vi "formal.vi"() -> ()   [LabVIEW 2011]
uses:
  <vilib>/Platform/storage/lvStorage.llb/_openFunction.ctl
  <vilib>/DAQmx/read.llb/DAQmx Read (Analog 1D Wfm NChan NSamp).vi
  <vilib>/Utility/file.llb/Write To Spreadsheet File (string).vi
  <vilib>/DAQmx/configure/timing.llb/DAQmx Timing (Sample Clock).vi
  <vilib>/Waveform/WDTOps.llb/WDT Index Channel DBL.vi
  <vilib>/Platform/storage/lvStorage.llb/_openStorageWithRootAutoDetect.vi
  <vilib>/Platform/storage/lvStorage.llb/xStorage/xStorageSupp/ErrorOut.vi
  <vilib>/Platform/storage/lvStorage.llb/_queryPropDateTime.vi
  <vilib>/Platform/storage/lvStorage.llb/_queryGenericObjects.vi
  <vilib>/Platform/storage/lvStorage.llb/_loadAllWaveform.vi
  <vilib>/Platform/storage/Storage.llb/Get Object Info.vi
  <vilib>/Platform/storage/Storage.llb/__closeStorageFromObject.vi
  <vilib>/DAQmx/calibration/calibrationInfo.llb/DAQmx Perform Shunt Calibration (Strain).vi
  <vilib>/DAQmx/miscellaneous.llb/DAQmx Fill In Error Info.vi
  <vilib>/Utility/file.llb/Write To Spreadsheet File (DBL).vi
  <vilib>/Platform/storage/lvStorage.llb/xStorage/Open Data Storage/Open Data Storage.xnode
  <vilib>/Platform/storage/lvStorage.llb/xStorage/Read Data/Read Data.xnode
  <vilib>/Platform/storage/lvStorage.llb/xStorage/Close Data Storage/Close Data Storage.xnode
  C:/Program Files (x86)/National Instruments/LabVIEW 2011/resource/objmgr/daqmx.rc
  <vilib>/Analysis/NI_AALBase.lvlib
panel:
  out "Working Folder":string="M:\\github\\DAQP"
  out "concatenated string":string="M:\\github\\DAQP\\_SP11_file_0.tdms"
  in  "stop":bool
  in  "voltage excitation source 2":i32(ring)=10200 items=["Internal"=10200, "External"=10167, "None"=10230]
  in  "voltage excitation source":i32(ring)=10200 items=["Internal"=10200, "External"=10167, "None"=10230]
  out "Config Flat Array":T1(array[cluster])=[{["234", "VoltageInputIntExc", "SC1mod1/ai0", "LVDT_5", "in."], "Voltage_cluster"={10.0, -10.0, 22.4, 0.0, TRUE, 60.0, 10.0}, "Strain_cluster"={0.0, 0.0, 0.0, 0.0, TRUE, 0.0, 0.0, 0.0, 0.0, ""}}, {["234424", "VoltageInputExtExc", "SC1mod1/ai1", "MTS_DISP_0_10_in", "in."], "Voltage_cluster"={10.0, -10.0, 22.4, 0.0, TRUE, 60.0, 0.4}, "Strain_cluster"={0.0, 0.0, 0.0, 0.0, TRUE, 0.0, 0.0, 0.0, 0.0, ""}}, {["1234", "StrainInput", "SC1mod1/ai2", "STRAIN_350_half", "microstrain"], "Voltage_cluster"={0.0, 0.0, 0.0, 0.0, TRUE, 0.0, 0.0}, "Strain_cluster"={0.01, -0.01, 1.0, 0.0, TRUE, 60.0, 3.125, 350.0, 2.0, "Half Bridge I"}}]
  out "Channel Indicator":i32[](array[numeric])=[2, 1, 0]
  out "Config Array":T1(array[cluster])=[{["234", "VoltageInputIntExc", "SC1mod1/ai0", "LVDT_5", "in."], "Voltage_cluster"={10.0, -10.0, 22.4, 0.0, TRUE, 60.0, 10.0}, "Strain_cluster"={0.0, 0.0, 0.0, 0.0, TRUE, 0.0, 0.0, 0.0, 0.0, ""}}, {["234424", "VoltageInputExtExc", "SC1mod1/ai1", "MTS_DISP_0_10_in", "in."], "Voltage_cluster"={10.0, -10.0, 22.4, 0.0, TRUE, 60.0, 0.4}, "Strain_cluster"={0.0, 0.0, 0.0, 0.0, TRUE, 0.0, 0.0, 0.0, 0.0, ""}}, {["1234", "StrainInput", "SC1mod1/ai2", "STRAIN_350_half", "microstrain"], "Voltage_cluster"={0.0, 0.0, 0.0, 0.0, TRUE, 0.0, 0.0}, "Strain_cluster"={0.01, -0.01, 1.0, 0.0, TRUE, 60.0, 3.125, 350.0, 2.0, "Half Bridge I"}}, {[], "Voltage_cluster"={0.0, 0.0, 0.0, 0.0, TRUE, 0.0, 0.0}, "Strain_cluster"={0.0, 0.0, 0.0, 0.0, TRUE, 0.0, 0.0, 0.0, 0.0, ""}}, {[], "Voltage_cluster"={0.0, 0.0, 0.0, 0.0, TRUE, 0.0, 0.0}, "Strain_cluster"={0.0, 0.0, 0.0, 0.0, TRUE, 0.0, 0.0, 0.0, 0.0, ""}}, {[], "Voltage_cluster"={0.0, 0.0, 0.0, 0.0, TRUE, 0.0, 0.0}, "Strain_cluster"={0.0, 0.0, 0.0, 0.0, TRUE, 0.0, 0.0, 0.0, 0.0, ""}}, {[], "Voltage_cluster"={0.0, 0.0, 0.0, 0.0, TRUE, 0.0, 0.0}, "Strain_cluster"={0.0, 0.0, 0.0, 0.0, TRUE, 0.0, 0.0, 0.0, 0.0, ""}}, {[], "Voltage_cluster"={0.0, 0.0, 0.0, 0.0, TRUE, 0.0, 0.0}, "Strain_cluster"={0.0, 0.0, 0.0, 0.0, TRUE, 0.0, 0.0, 0.0, 0.0, ""}}, {[], "Voltage_cluster"={0.0, 0.0, 0.0, 0.0, TRUE, 0.0, 0.0}, "Strain_cluster"={0.0, 0.0, 0.0, 0.0, TRUE, 0.0, 0.0, 0.0, 0.0, ""}}, {[], "Voltage_cluster"={0.0, 0.0, 0.0, 0.0, TRUE, 0.0, 0.0}, "Strain_cluster"={0.0, 0.0, 0.0, 0.0, TRUE, 0.0, 0.0, 0.0, 0.0, ""}}, {[], "Voltage_cluster"={0.0, 0.0, 0.0, 0.0, TRUE, 0.0, 0.0}, "Strain_cluster"={0.0, 0.0, 0.0, 0.0, TRUE, 0.0, 0.0, 0.0, 0.0, ""}}, {[], "Voltage_cluster"={0.0, 0.0, 0.0, 0.0, TRUE, 0.0, 0.0}, "Strain_cluster"={0.0, 0.0, 0.0, 0.0, TRUE, 0.0, 0.0, 0.0, 0.0, ""}}, {[], "Voltage_cluster"={0.0, 0.0, 0.0, 0.0, TRUE, 0.0, 0.0}, "Strain_cluster"={0.0, 0.0, 0.0, 0.0, TRUE, 0.0, 0.0, 0.0, 0.0, ""}}, {[], "Voltage_cluster"={0.0, 0.0, 0.0, 0.0, TRUE, 0.0, 0.0}, "Strain_cluster"={0.0, 0.0, 0.0, 0.0, TRUE, 0.0, 0.0, 0.0, 0.0, ""}}, {[], "Voltage_cluster"={0.0, 0.0, 0.0, 0.0, TRUE, 0.0, 0.0}, "Strain_cluster"={0.0, 0.0, 0.0, 0.0, TRUE, 0.0, 0.0, 0.0, 0.0, ""}}, {[], "Voltage_cluster"={0.0, 0.0, 0.0, 0.0, TRUE, 0.0, 0.0}, "Strain_cluster"={0.0, 0.0, 0.0, 0.0, TRUE, 0.0, 0.0, 0.0, 0.0, ""}}, {[], "Voltage_cluster"={0.0, 0.0, 0.0, 0.0, TRUE, 0.0, 0.0}, "Strain_cluster"={0.0, 0.0, 0.0, 0.0, TRUE, 0.0, 0.0, 0.0, 0.0, ""}}, {[], "Voltage_cluster"={0.0, 0.0, 0.0, 0.0, TRUE, 0.0, 0.0}, "Strain_cluster"={0.0, 0.0, 0.0, 0.0, TRUE, 0.0, 0.0, 0.0, 0.0, ""}}, {[], "Voltage_cluster"={0.0, 0.0, 0.0, 0.0, TRUE, 0.0, 0.0}, "Strain_cluster"={0.0, 0.0, 0.0, 0.0, TRUE, 0.0, 0.0, 0.0, 0.0, ""}}, {[], "Voltage_cluster"={0.0, 0.0, 0.0, 0.0, TRUE, 0.0, 0.0}, "Strain_cluster"={0.0, 0.0, 0.0, 0.0, TRUE, 0.0, 0.0, 0.0, 0.0, ""}}, {[], "Voltage_cluster"={0.0, 0.0, 0.0, 0.0, TRUE, 0.0, 0.0}, "Strain_cluster"={0.0, 0.0, 0.0, 0.0, TRUE, 0.0, 0.0, 0.0, 0.0, ""}}, {[], "Voltage_cluster"={0.0, 0.0, 0.0, 0.0, TRUE, 0.0, 0.0}, "Strain_cluster"={0.0, 0.0, 0.0, 0.0, TRUE, 0.0, 0.0, 0.0, 0.0, ""}}, {[], "Voltage_cluster"={0.0, 0.0, 0.0, 0.0, TRUE, 0.0, 0.0}, "Strain_cluster"={0.0, 0.0, 0.0, 0.0, TRUE, 0.0, 0.0, 0.0, 0.0, ""}}, {[], "Voltage_cluster"={0.0, 0.0, 0.0, 0.0, TRUE, 0.0, 0.0}, "Strain_cluster"={0.0, 0.0, 0.0, 0.0, TRUE, 0.0, 0.0, 0.0, 0.0, ""}}, {[], "Voltage_cluster"={0.0, 0.0, 0.0, 0.0, TRUE, 0.0, 0.0}, "Strain_cluster"={0.0, 0.0, 0.0, 0.0, TRUE, 0.0, 0.0, 0.0, 0.0, ""}}, {[], "Voltage_cluster"={0.0, 0.0, 0.0, 0.0, TRUE, 0.0, 0.0}, "Strain_cluster"={0.0, 0.0, 0.0, 0.0, TRUE, 0.0, 0.0, 0.0, 0.0, ""}}, {[], "Voltage_cluster"={0.0, 0.0, 0.0, 0.0, TRUE, 0.0, 0.0}, "Strain_cluster"={0.0, 0.0, 0.0, 0.0, TRUE, 0.0, 0.0, 0.0, 0.0, ""}}, {[], "Voltage_cluster"={0.0, 0.0, 0.0, 0.0, TRUE, 0.0, 0.0}, "Strain_cluster"={0.0, 0.0, 0.0, 0.0, TRUE, 0.0, 0.0, 0.0, 0.0, ""}}, {[], "Voltage_cluster"={0.0, 0.0, 0.0, 0.0, TRUE, 0.0, 0.0}, "Strain_cluster"={0.0, 0.0, 0.0, 0.0, TRUE, 0.0, 0.0, 0.0, 0.0, ""}}, {[], "Voltage_cluster"={0.0, 0.0, 0.0, 0.0, TRUE, 0.0, 0.0}, "Strain_cluster"={0.0, 0.0, 0.0, 0.0, TRUE, 0.0, 0.0, 0.0, 0.0, ""}}, {[], "Voltage_cluster"={0.0, 0.0, 0.0, 0.0, TRUE, 0.0, 0.0}, "Strain_cluster"={0.0, 0.0, 0.0, 0.0, TRUE, 0.0, 0.0, 0.0, 0.0, ""}}, {[], "Voltage_cluster"={0.0, 0.0, 0.0, 0.0, TRUE, 0.0, 0.0}, "Strain_cluster"={0.0, 0.0, 0.0, 0.0, TRUE, 0.0, 0.0, 0.0, 0.0, ""}}]
  in  "Tab Control":T2(tab)=enum."check Fatigue tdms file"
  in  "SXCI Chassis Name":string="/SC1"
  in  "Config File Path":path=path "M:/github/DAQP/xml_temp.xml"
  in  "Task Name":refnum<k21>="new Task"
  in  "custom scale name":tag="linear1"
  in  "error in":errorcluster
  out "Total Number of Channel in Use":i32=3
  in  "Go Button":bool
  out "Utility Usage Array":cluster{bool, string}[][](array[cluster])=[[{TRUE, "234"}, {FALSE, ""}, {FALSE, ""}, {FALSE, ""}], [{TRUE, "234424"}, {FALSE, ""}, {FALSE, ""}, {FALSE, ""}], [{TRUE, "1234"}, {FALSE, ""}, {FALSE, ""}, {FALSE, ""}], [{FALSE, ""}, {FALSE, ""}, {FALSE, ""}, {FALSE, ""}], [{FALSE, ""}, {FALSE, ""}, {FALSE, ""}, {FALSE, ""}], [{FALSE, ""}, {FALSE, ""}, {FALSE, ""}, {FALSE, ""}], [{FALSE, ""}, {FALSE, ""}, {FALSE, ""}, {FALSE, ""}], [{FALSE, ""}, {FALSE, ""}, {FALSE, ""}, {FALSE, ""}]]
  in  "Measure actual excitation?":bool
  in  "Shunt Resistance":dbl=100000.0 format="%0.2f"
  in  "Shunt Location":enum32{"R1", "R2", "R3", "R4"}(ring)=enum."R3"
  in  "error out":errorcluster
  in  "sample rate":dbl=1000.0
  in  "number of samples per channel (buffer size)":i32=10000000
  in  "number of samples per channel":i32=200
  in  "Offset Nulling":bool
  in  "Display Channel":u16(ring)=1 items=["234", "234424", "1234"]
  out "Display Channel results":dbl[](graph)=[22.61393258426966] caption="Real Time Data Acquision Chart"
  out "Result Array":dbl[](array[numeric])=[3.695945285784074, 22.61393258426966, -0.0019209204014080854]
  out "Strain Channel Name":string[](array[string])=["1234"]
  out "Channel Physical Name":string[](array[string])=["SC1mod1/ai0", "SC1mod1/ai1", "SC1mod1/ai2"]
  out "Channel Name Array":string[](array[string])=["234", "234424", "1234"]
  out "Channel Unit Array":string[](array[string])=["in.", "in.", "microstrain"]
  out "Factor A":dbl[](array[numeric])=[22.4, 22.4, 1.0]
  out "Factor B":dbl[](array[numeric])
  out "Factor N":dbl[](array[numeric])
  in  "Start DAQ":bool=TRUE
  in  "shunt":bool
  out "LVM result file path":path=path "M:/github/DAQP/trial_newnew.lvm"
  out "AvailSampPerChan":u32=9
  in  "Start Recording":bool
  out "Csv Result File":path=path "M:/github/DAQP/trial_newnew.txt"
  in  "Record File Path":string="trial_newnew"
  in  "Start Fatigue Module":bool=TRUE
  in  "Recording cycles (M)":i32=5
  in  "Recording interval (N)":i32=10
  out "Cycle count measuring":string="234"
  in  "Name of specimen":string="_SP11"
  in  "Lowerbound":dbl=-4.6
  in  "Upbond":dbl=4.6
  in  "Channel to count cycle":i32
  out "Fatigue data recording in progress":bool=TRUE
  out "Valley":bool
  out "Peak":bool=TRUE
  out "Current cycle numbers":dbl
  in  "Start Cycle":i32
  in  "file path":path=path "C:/Documents and Settings/ju112496/Desktop/seminar/seminar1_SP11_file_30.tdms"
  out "Total Channel numbers":i32=3
  in  "Display channel":i32
  out "Display Channel name":string="potential meter"
  in  "Load file":bool
  out "Waveform Graph":waveform(dbl)(graph)={"t0"=timestamp(3600 s since 1904-01-01), "dt"=1.0, "Y"=[4.96518220736595, 4.9879295957189544, 4.987880843319572, 4.9878564031395225, 4.98785639543025, 4.98785639543025, 4.987880804692245, 4.9878563940215805, 4.9878960256751075, 4.987890269213241, 4.987881073821511, 4.987880252277753, 4.987929618872902, 4.987856395547572, 4.98788080318033, 4.987856395533495, 4.987880803283583, 4.987906295992125, 4.98787971833429, 4.9878586312981446, 4.987878567509733, 4.987856395430245, 4.98785639543025, 4.98785639543025, 4.98785639543025, 4.987883590063237, 4.987878016503915, 4.98788151128357, 4.987855687430249, 4.98785639543025, 4.987929617963517, 4.9878563964569524, 4.987880803283373, 4.987856395430452, 4.98785639543025, 4.98785639543025, 4.98788084098527, 4.987880765581879, 4.987931213533417, 4.987879208800789, 4.987930169857925, 4.987855844502128, 4.987874416787948, 4.987880803283574, 4.987935976028989, 4.9879052089034515, 4.987954058719019, 4.9847496503819215, 2.892462538878111, -2.2229287425946533, -4.973634617887958, -5.002277969332104, -5.0022779693255774, -5.0022779693255774, -5.001646607827787, -0.31893796746551445, 4.632149520376136, 4.98790575411758, 4.98792911085913, 4.9878808211186305, 4.98788080338445, 4.987929900245035, 4.987904929884249, 4.698784785906143, 0.9667412484497627, -3.879258099878396, -5.002259664842451, -5.00227796932558, -5.0022779693255774, -5.0022779693255774, -5.0022779693255774, -1.4532621065694493, 4.4686316784738045, 4.987856401837168, 4.987905209618321, 4.987871617931691, 4.987898537146574, 3.702899980763011, 0.06222091586554777, -3.748607068444104, -5.002254326371235, -5.002277969325581, -5.0022779693255774, -4.374557750317882, 2.8051749196435076, 4.987837636717955, 4.987881293140786, 4.987904721229926, 4.987880802998693, 4.973936289936798, 2.657868551030198, -2.141567304353255, -4.984397753147493, -5.002277969328984, -5.0022779693255774, -4.964414117866688, -0.8359451058702335, 4.556547925816468, 4.987905212444337, 4.987905179546101, 4.9878564270125985, 4.98785639543025, 4.914856957749751, 2.6205127878625833, -2.157142345502778, -4.966675154023192, -5.002277969332567, -5.0022779693255774, -5.0022779693255774, -4.996944784883012, -1.1325883571495219, 4.482358752630597], "attributes"=variant("NI_ChannelName"=variant(string "Untitled"), "NI_UnitDescription"=variant(string ""))}
  # "Sampling rate setting"
  # "Shunt Calibration information"
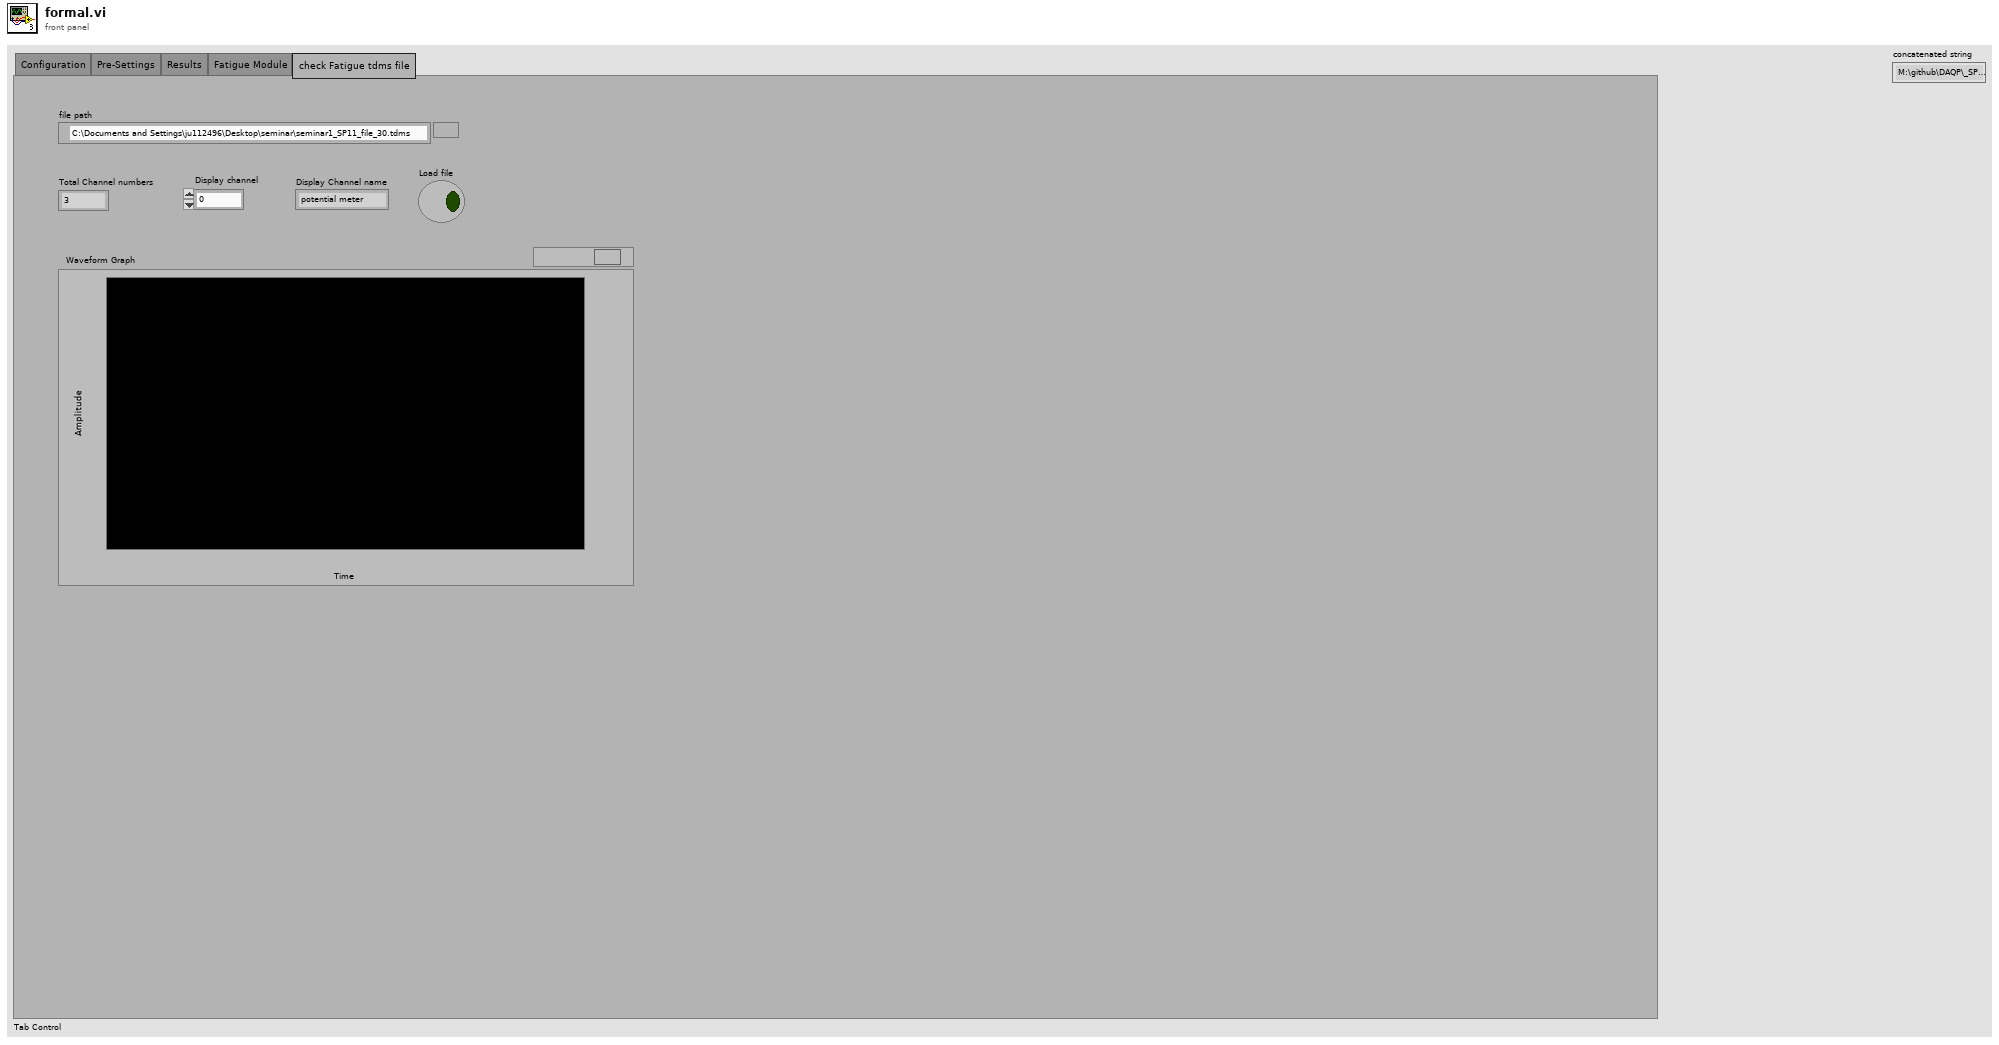
[diagram p1: front panel]
types:
  T1 = cluster{string[], "Voltage_cluster":cluster{dbl, dbl, dbl, dbl, bool, dbl, dbl}, "Strain_cluster":cluster{dbl, dbl, dbl, dbl, bool, dbl, dbl, dbl, dbl, string}}[]
  T2 = enum32{"Configuration", "Pre-Settings", "Results", "Fatigue Module", "check Fatigue tdms file"}
  T3 = enum16{"UPDATE", "READ", "QUERY", "CREATE CHILD", "CREATE", "CONNECT", "DISCONNECT"}
  T4 = typedef "_openFunction.ctl" = enum16{"open", "open or create", "create or replace", "create", "open (read only)"}
  T5 = cluster{dbl, dbl, dbl, dbl, bool, dbl, dbl, dbl, dbl, string}
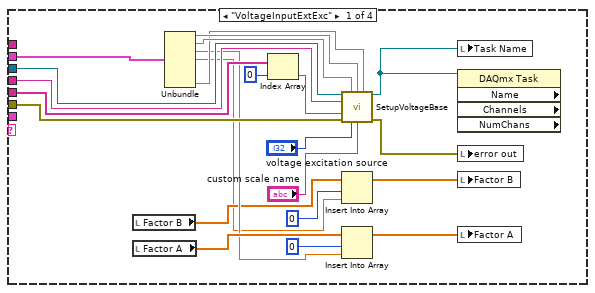
[diagram p3: hidden frame]
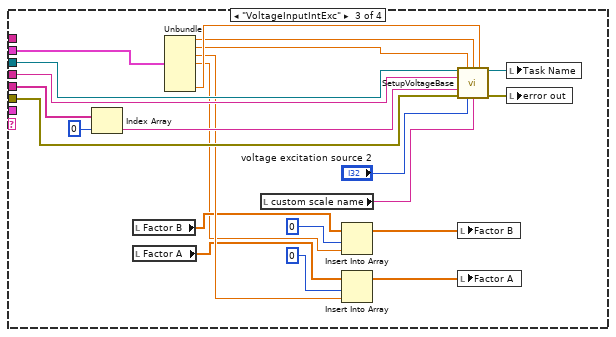
[diagram p5: hidden frame]
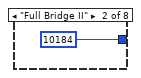
[diagram p6: hidden frame]
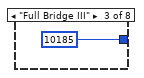
[diagram p7: hidden frame]
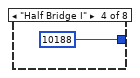
[diagram p8: hidden frame]
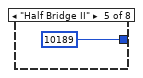
[diagram p9: hidden frame]
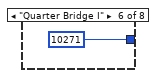
[diagram p10: hidden frame]
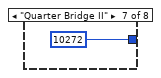
[diagram p11: hidden frame]
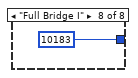
[diagram p12: hidden frame]
diagram:
  # "Step 5: Main DAQ Loop"
  # "Step 4: Add channel to task, based on the type and input parameters"
  # "Step 3: Generate flatted channel settings and initialize factors"
  # "Step 2: Scan Setting config file and build in use channel array, show channel in use array on front panel"
  # "Step 1: Specify config file and initialize variables"
  n1 = flat-sequence {
    tunnel: [w16] -> w2
    tunnel: w2 -> [_]
    tunnel: [w84] -> w1
    tunnel: w1 -> [_]
    frame #0 {
      w3 = FALSE
      # "Wait unitl sepcify the config file"
      # "Control of start fatigue detection module"
      # "Control of Start data save to file"
      # "Control Start of DAQ process"
      n2 = local write "Start DAQ"(w3) -> ()
      n3 = local write "Start Fatigue Module"(w3) -> ()
      n4 = local write "Start Recording"(w3) -> ()
      n5 = for {
        N: 32 -> [_]
        tunnel: [w17] -> w10 mode=indexing
        n6 = Bundle(FALSE, "") -> (w17:cluster{bool, string})  [unwired: 1 in]
      }
      n7 = Initialize Array("", 0 ("dimension size")) -> (→"Channel Name Array":string[])
      n8 = Reshape Array(w10, 4 ("dimension size"), 8 ("dimension size")) -> (w12:cluster{bool, string}[][])
      n9 = while {
        tunnel: ["Go Button"] -> w16
        stop <- "Go Button" stop-if-true
        n10 = Wait (ms)(milliseconds to wait=u32 500) -> ()  [unwired: 1 out]
      }
      n11 = Transpose 2D Array(2D array=w12) -> (transposed array=→"Utility Usage Array":cluster{bool, string}[][])
      n12 = Initialize Array(0.0 ("element")) -> (w5:dbl[])  [unwired: 1 in]
      n13 = local write "Display Channel results"(w5) -> ()
      "Total Number of Channel in Use" <- 0 ("Total Number of Channel in Use")
    }
    frame #1 {
      w36 = 0 ("dimension size")
      n14 = Initialize Array("", 0 ("dimension size")) -> (→"Strain Channel Name":string[])
      n15 = Initialize Array(0.0, 0 ("dimension size")) -> (→"Factor A":dbl[])
      n16 = Initialize Array(0.0, 0 ("dimension size")) -> (→"Factor B":dbl[])
      n17 = Initialize Array(w36, w36) -> (→"Channel Indicator":i32[])
      n18 = local read "Config File Path"() -> (w35:path)
      n19 = Read from Text File(file (use dialog)=w35) -> (text=w43:string)  [unwired: 3 in, 3 out]
      n20 = call "importxml.vi"("String"=w43, "sc"="SXCI Chassis Name") -> ("output array"=w38:T1)  [unwired: 9 in]
      "Config Array" <- w38
      n21 = for {
        tunnel: w38 -> [w54] mode=indexing
        tunnel: [w47] -> w39 mode=indexing
        i -> [w45]
        w52 = 0 ("index")
        n22 = Unbundle(w54) -> (w49:string[])  [unwired: 2 out]
        n23 = Index Array(array=w49, index=w52) -> (element=w53:string)
        n24 = String Length(string=w53) -> (length=w51:i32)
        n25 = Index Array(array=w49, index=0) -> (element=w48:string)
        n26 = Greater?(x=w51, y=w52) -> (0:w46:bool)
        n27 = Bundle(w46, w48) -> (w47:cluster{bool, string})  [unwired: 1 in]
        n28 = case shown="True" w46 {
          tunnel: w45 -> [_ w58]
          frame False {
          }
          frame True {
            n29 = local read "Channel Indicator"() -> (w56:i32[])
            n30 = Insert Into Array(array=w56, index=0, new element=w58) -> (w55:i32[])
            n31 = local write "Channel Indicator"(w55) -> ()
          }
        }
      }
      n32 = local read "Config File Path"() -> (w24:path)
      n33 = Strip Path(path=w24) -> (stripped path=w23:path)  [unwired: 1 out]
      n34 = Path To String(path=w23) -> (string=→"Working Folder":string)
      n35 = Reshape Array(w39, 4 ("dimension size"), 8 ("dimension size")) -> (w40:cluster{bool, string}[][])
      n36 = Transpose 2D Array(2D array=w40) -> (transposed array=w25:cluster{bool, string}[][])
      n37 = local write "Utility Usage Array"(w25) -> ()
    }
    frame #2 {
      n38 = local read "Channel Indicator"() -> (w66:i32[])
      n39 = Reverse 1D Array(array=w66) -> (reversed array=w69:i32[])
      n40 = for {
        tunnel: w69 -> [w71] mode=indexing
        tunnel: [w72] -> w65 mode=indexing
        n41 = local read "Config Array"() -> (w73:T1)
        n42 = Array Subset(array=w73, index=w71, length=1) -> (w72:T1)
      }
      n43 = Array Size(array=w65) -> (size(s)=w68:i32[])
      n44 = Index Array(array=w68, index=0) -> (element=w59:i32)
      n45 = local write "Total Number of Channel in Use"(w59) -> ()
      n46 = Reshape Array(w65, w59) -> (→"Config Flat Array":T1)
      n47 = Initialize Array(0.0 ("element"), w59) -> (→"Factor N":dbl[])
      n48 = Initialize Array(0.0 ("element"), w59) -> (→"Result Array":dbl[])
    }
    frame #3 {
      w93 = TRUE  # auto cleanup
      # "Initialize the result output files"
      n49 = local read "Total Number of Channel in Use"() -> (w87:i32)
      n50 = local read "Config Flat Array"() -> (w89:T1)
      n51 = local read "Working Folder"() -> (w74:string)
      n52 = call <vilib>:"DAQmx Create Task.vi"("new task name"="new Task", "auto cleanup"=w93, "error in"="error in") -> ("task out"=w91:refnum<k21>, "error out"=w90:errorcluster)  [unwired: 2 in, 9 out]
      n53 = for {
        N: w87 -> [_]
        tunnel: w89 -> [w110] mode=indexing
        tunnel: w91 -> [w108]
        tunnel: w90 -> [w107]
        tunnel: [w99] -> w88 mode=indexing
        tunnel: [w100] -> w86 mode=indexing
        tunnel: [w97] -> w85 mode=indexing
        n54 = Unbundle(w110) -> (w102:string[], "Voltage_cluster"=w106:cluster{dbl, dbl, dbl, dbl, bool, dbl, dbl}, "Strain_cluster"=w103:T5)
        n55 = Index Array(array=w102, index=0) -> (element=w99:string)
        n56 = Index Array(array=w102, index=2) -> (element=w97:string)
        n57 = Index Array(array=w102, index=1) -> (element=w98:string)
        n58 = Index Array(array=w102, index=4) -> (element=w100:string)
        n59 = case shown="\"StrainInput\"" w98 {
          tunnel: w108 -> [w128 _ w152 w174]
          tunnel: w107 -> [w127 _ w151 w173]
          tunnel: w106 -> [w126 _ w153 _]
          tunnel: w102 -> [w125 _ w150 _]
          tunnel: w97 -> [w120 _ w142 w167]
          tunnel: w103 -> [_ _ _ w180]
          tunnel: w99 -> [_ _ _ w166]
          frame "VoltageInputExtExc" {
            n60 = local read "Factor B"() -> (w114:dbl[])
            n61 = local read "Factor A"() -> (w117:dbl[])
            n62 = Unbundle(w126) -> (w131:dbl, w130:dbl, w115:dbl, w112:dbl, w121:dbl)  [unwired: 2 out]
            n63 = Index Array(array=w125, index=0) -> (element=w119:string)
            n64 = call "SetupVoltageBase.vi"("Refnum in"=w128, "min"=w130, "max"=w131, "excitation value"=w121, "physical channel"=w120, "String"=w119, "error in (no error)"=w127, "voltage excitation source"="voltage excitation source", "custom scale name"="custom scale name") -> ("Refnum out"=w122:refnum<k21>, "error out"=w123:errorcluster)  [unwired: 5 in]
            n65 = Insert Into Array(array=w114, index=0, new element=w112) -> (w111:dbl[])
            n66 = Insert Into Array(array=w117, index=0, new element=w115) -> (w116:dbl[])
            n67 = local write "Task Name"(w122) -> ()
            n68 = property class="DAQmx Task" props=["Name", "Channels", "NumChans"](reference=w122) -> ()  [unwired: 1 in, 5 out]
            n69 = local write "error out"(w123) -> ()
            n70 = local write "Factor B"(w111) -> ()
            n71 = local write "Factor A"(w116) -> ()
          }
          frame "Null", Default {
          }
          frame "VoltageInputIntExc" {
            n72 = Index Array(array=w150, index=0) -> (element=w141:string)
            n73 = local read "Factor B"() -> (w135:dbl[])
            n74 = local read "Factor A"() -> (w138:dbl[])
            n75 = Unbundle(w153) -> (w144:dbl, w143:dbl, w140:dbl, w134:dbl, w149:dbl)  [unwired: 2 out]
            n76 = local read "custom scale name"() -> (w148:tag)
            n77 = Insert Into Array(array=w135, index=0, new element=w134) -> (w133:dbl[])
            n78 = Insert Into Array(array=w138, index=0, new element=w140) -> (w137:dbl[])
            n79 = call "SetupVoltageBase.vi"("Refnum in"=w152, "min"=w143, "max"=w144, "excitation value"=w149, "physical channel"=w142, "String"=w141, "error in (no error)"=w151, "voltage excitation source"="voltage excitation source 2", "custom scale name"=w148) -> ("Refnum out"=w146:refnum<k21>, "error out"=w145:errorcluster)  [unwired: 5 in]
            n80 = local write "Factor B"(w133) -> ()
            n81 = local write "Factor A"(w137) -> ()
            n82 = local write "Task Name"(w146) -> ()
            n83 = local write "error out"(w145) -> ()
          }
          frame "StrainInput" {
            n84 = Unbundle(w180) -> (w179:dbl, w178:dbl, w159:dbl, w156:dbl, w177:dbl, w176:dbl, w175:dbl, w169:string)  [unwired: 2 out]
            n85 = local read "Factor B"() -> (w158:dbl[])
            n86 = local read "Factor A"() -> (w160:dbl[])
            n87 = case shown="\"Null\", Default" w169 {
              tunnel: [0 10184 10185 10188 10189 10271 10272 10183] -> w168
              frame "Null", Default {
              }
              frame "Full Bridge II" {
              }
              frame "Full Bridge III" {
              }
              frame "Half Bridge I" {
              }
              frame "Half Bridge II" {
              }
              frame "Quarter Bridge I" {
              }
              frame "Quarter Bridge II" {
              }
              frame "Full Bridge I" {
              }
            }
            n88 = local read "Strain Channel Name"() -> (w164:string[])
            n89 = local read "custom scale name"() -> (w172:tag)
            n90 = Insert Into Array(array=w158, index=0, new element=w156) -> (w155:dbl[])
            n91 = Insert Into Array(array=w160, index=0, new element=w159) -> (w161:dbl[])
            n92 = call "SetupStrainBase.vi"("Refnum in"=w174, "excitation value"=w177, "physical channel"=w167, "channel name"=w166, "minimum value"=w178, "nominal gage resistance"=w176, "maximum value"=w179, "error in (no error)"=w173, "custom scale name"=w172, "gage factor"=w175, "strain configuration"=w168) -> ("Refnum out"=w171:refnum<k21>, "error out"=w170:errorcluster)  [unwired: 3 in]
            n93 = local write "Factor B"(w155) -> ()
            n94 = local write "Factor A"(w161) -> ()
            n95 = Insert Into Array(array=w164, index=0, new element=w166) -> (w163:string[])
            n96 = local write "error out"(w170) -> ()
            n97 = local write "Strain Channel Name"(w163) -> ()
            n98 = local write "Task Name"(w171) -> ()
          }
        }
      }
      "Channel Unit Array" <- w86
      "Channel Physical Name" <- w85
      n99 = Concatenate Strings(w74, "\\" ("string"), "Record File Path", ".txt" ("string")) -> (w83:string)
      n100 = Concatenate Strings(w74, "\\" ("string"), "Record File Path", ".lvm") -> (w81:string)
      n101 = String To Path(string=w81) -> (path=→"LVM result file path":path)
      n102 = String To Path(string=w83) -> (path=→"Csv Result File":path)
      n103 = while {
        tunnel: [w95] -> w84
        stop <- w95 stop-if-true
        n104 = local read "Start DAQ"() -> (w95:bool)
        n105 = Wait (ms)(milliseconds to wait=u32 500) -> ()  [unwired: 1 out]
      }
      n106 = local write "Channel Name Array"(w88) -> ()
    }
    frame #4 {
      w208 = 10123 items=["Finite Samples"=10178, "Continuous Samples"=10123, "Hardware Timed Single Point"=12522]  # sample mode
      # "Step 5.1 Sampling rate Set"
      # "Add head to the csv output file, column header and unit"
      n107 = local read "Channel Name Array"() -> (w197:string[])
      n108 = case shown="True" "Load file" {
        frame False {
        }
        frame True {
          n109 = local write "Load file"(FALSE ("Load file")) -> ()
          n110 = xnode "Open Data Storage\n[TDMS]"("file path"="file path") -> ("storage refnum (file)"=w218:refnum<k20>)  [unwired: 2 in, 4 out]
          n111 = local read "Channel Name Array"() -> (w213:string[])
          n112 = xnode "Read Data\n[Channel]"("storage refnum (file)"=w218) -> ("Signal"=w214:waveform(dbl)[], "storage refnum (file) out"=w219:refnum<k20>)  [unwired: 3 out]
          n113 = xnode "Close Data Storage\n"("storage refnum (file)"=w219) -> ()  [unwired: 3 out]
          n114 = Array Size(array=w214) -> (size(s)=→"Total Channel numbers":i32)
          n115 = Index Array(array=w213, index="Display channel") -> (element=→"Display Channel name":string)
          n116 = call-poly <vilib>:"Index Waveform Array.vi"("index"="Display channel", "waveform array"=w214) -> ("waveform"=→"Waveform Graph":waveform(dbl))  [unwired: 1 in, 8 out]
        }
      }
      n117 = local read "Factor A"() -> (w201:dbl[])
      n118 = local read "Factor B"() -> (w199:dbl[])
      n119 = local write "Current cycle numbers"("Start Cycle") -> ()
      n120 = Reverse 1D Array(array=w201) -> (reversed array=w200:dbl[])
      n121 = Reverse 1D Array(array=w199) -> (reversed array=w198:dbl[])
      n122 = local write "Factor A"(w200) -> ()
      n123 = local write "Factor B"(w198) -> ()
      n124 = property on="Display Channel" class="Ring (strict)"("Strings []"=w197) -> ()  [unwired: 2 in, 2 out]
      n125 = local read "Task Name"() -> (w205:refnum<k21>)
      n126 = local read "error out"() -> (w204:errorcluster)
      n127 = local read "Channel Name Array"() -> (w196:string[])
      n128 = local read "Channel Unit Array"() -> (w193:string[])
      n129 = local read "Csv Result File"() -> (w191:path)
      n130 = call <vilib>:"DAQmx Unflatten Channel String.vi"("names in"=w205) -> ()  [unwired: 1 in, 14 out]
      n131 = Build Array(w196, w193) -> (w192:string[][])
      n132 = call-poly <vilib>:"DAQmx Timing.vi"("task/channels in"=w205, "sample mode"=w208, "samples per channel"="number of samples per channel (buffer size)", "rate"="sample rate", "error in"=w204) -> ("task out"=w207:refnum<k21>, "error out"=w206:errorcluster)  [unwired: 2 in, 7 out]
      n133 = call-poly <vilib>:"Write To Spreadsheet File.vi"("delimiter (\\t)"="," ("delimiter (\\t)"), "append to file? (new file:F)"=FALSE, "2D data"=w192, "file path (dialog if empty)"=w191) -> ()  [unwired: 4 in, 1 out]
      n134 = call <vilib>:"DAQmx Start Task.vi"("task/channels in"=w207, "error in"=w206) -> ("task out"=w203:refnum<k21>, "error out"=w202:errorcluster)  [unwired: 12 out]
      n135 = while {
        tunnel: w203 -> [w258]
        tunnel: w202 -> [w257]
        stop <- "stop" stop-if-true
        # "Step 5.3  Data averaging and save to csv file for static test"
        # "Step 5.2  Nulling (hardware/offshift/shunt calibration) based on the switchers and request"
        n136 = flat-sequence {
          tunnel: [w260] -> w256
          tunnel: [w259] -> w255
          tunnel: w258 -> [w262]
          tunnel: w257 -> [w261]
          tunnel: w256 -> [w350]
          tunnel: w255 -> [w349]
          tunnel: [w339] -> w253
          tunnel: w253 -> [w378]
          frame #0 {
            n137 = case shown="True" "Offset Nulling" {
              tunnel: w262 -> [w265 w276]
              tunnel: w261 -> [w264 w275]
              tunnel: [w265 w274] -> w260
              tunnel: [w264 w273] -> w259
              frame False {
              }
              frame True {
                # "Restart the daq"
                # "Adjust Max and Min based on the reading of voltage values"
                # "Do Shunt Calibration"
                # "Do hardware Nulling"
                n138 = flat-sequence {
                  tunnel: w276 -> [w278]
                  tunnel: [w281] -> w270
                  tunnel: [w280] -> w268
                  tunnel: w275 -> [w279]
                  tunnel: [w277] -> w266
                  tunnel: w270 -> [w289]
                  tunnel: [w287] -> w269
                  tunnel: w268 -> [w288]
                  tunnel: [w286] -> w267
                  tunnel: w266 -> [w290]
                  tunnel: w269 -> [w304]
                  tunnel: w267 -> [w303]
                  tunnel: [w302] -> w272
                  tunnel: [w301] -> w271
                  tunnel: w272 -> [w313]
                  tunnel: w271 -> [w312]
                  tunnel: [w335] -> w273
                  tunnel: [w336] -> w274
                  frame #0 {
                    n139 = local read "Strain Channel Name"() -> (w284:string[])
                    n140 = call <vilib>:"DAQmx Flatten Channel String.vi"("names in"=w284) -> ("names out"=w277:string)  [unwired: 1 in, 13 out]
                    n141 = call <vilib>:"DAQmx Stop Task.vi"("task/channels in"=w278, "error in"=w279) -> ("task out"=w282:refnum<k21>, "error out"=w283:errorcluster)  [unwired: 12 out]
                    n142 = call <vilib>:"DAQmx Perform Bridge Offset Nulling Calibration.vi"("task/channels in"=w282, "channels"=w277, "error in"=w283) -> ("task out"=w281:refnum<k21>, "error out"=w280:errorcluster)  [unwired: 1 in, 10 out]
                  }
                  frame #1 {
                    n143 = case shown="True" "shunt" {
                      tunnel: w290 -> [_ w297]
                      tunnel: w289 -> [w292 w296]
                      tunnel: w288 -> [w291 w295]
                      tunnel: [w292 w294] -> w287
                      tunnel: [w291 w293] -> w286
                      frame False {
                      }
                      frame True {
                        n144 = call-poly <vilib>:"DAQmx Perform Shunt Calibration.vi"("task/channels in"=w296, "channels"=w297, "shunt resistance"="Shunt Resistance", "shunt element location"="Shunt Location", "error in"=w295, "skip unsupported channels"=TRUE) -> ("task out"=w294:refnum<k21>, "error out"=w293:errorcluster)  [unwired: 8 in]
                      }
                    }
                  }
                  frame #2 {
                    n145 = call <vilib>:"DAQmx Start Task.vi"("task/channels in"=w304, "error in"=w303) -> ("task out"=w302:refnum<k21>, "error out"=w301:errorcluster)  [unwired: 12 out]
                  }
                  frame #3 {
                    # "Get Average voltage readings"
                    n146 = call-poly <vilib>:"DAQmx Read.vi"("task/channels in"=w313, "number of samples per channel"=1000, "error in"=w312) -> ("task out"=w308:refnum<k21>, "data"=w307:waveform(dbl)[], "error out"=w309:errorcluster)  [unwired: 10 in]
                    n147 = call <vilib>:"DAQmx Stop Task.vi"("task/channels in"=w308, "error in"=w309) -> ("task out"=w306:refnum<k21>)  [unwired: 12 in, 1 out]
                    n148 = for {
                      tunnel: w307 -> [w334] mode=indexing
                      tunnel: [w333] -> _ mode=indexing
                      tunnel: [w333] -> _ mode=indexing
                      tunnel: [w333] -> w310 mode=indexing
                      n149 = call <vilib>:"Mean.vi"("X"=w334) -> ("mean"=w333:dbl)  [unwired: 1 out]
                    }
                    n150 = local read "Channel Name Array"() -> (w305:string[])
                    n151 = for {
                      tunnel: w310 -> [w324] mode=indexing
                      tunnel: w306 -> [w323]
                      tunnel: w305 -> [w322] mode=indexing
                      w316 = -10.0 ("y")
                      w320 = 10.0 ("y")
                      n152 = property class="DAQmx Channel"(reference=w323, "ActiveChans"=w322) -> (reference out=w328:refnum<k21>, error out=w327:errorcluster, "AI.Max"=w326:dbl, "AI.Min"=w325:dbl)  [unwired: 1 in]
                      n153 = Add(x=w326, y=w324) -> (x+y=w318:dbl)
                      n154 = Add(x=w325, y=w324) -> (x+y=w315:dbl)
                      n155 = Greater Or Equal?(x=w318, y=w320) -> (x >= y?=w321:bool)
                      n156 = Less Or Equal?(x=w315, y=w316) -> (x <= y?=w317:bool)
                      n157 = case shown="True" w321 {
                        tunnel: w320 -> [_ w332]
                        tunnel: [w331 w332] -> w319
                        tunnel: w318 -> [w331 _]
                        frame False {
                        }
                        frame True {
                        }
                      }
                      n158 = case shown="True" w317 {
                        tunnel: w316 -> [_ w330]
                        tunnel: [w329 w330] -> w314
                        tunnel: w315 -> [w329 _]
                        frame False {
                        }
                        frame True {
                        }
                      }
                      n159 = property class="DAQmx Channel"(reference=w328, error in=w327, "ActiveChans"=w322, "AI.Max"=w319, "AI.Min"=w314) -> ()  [unwired: 2 out]
                    }
                  }
                  frame #4 {
                    n160 = local read "Task Name"() -> (w338:refnum<k21>)
                    n161 = local read "error out"() -> (w337:errorcluster)
                    n162 = call <vilib>:"DAQmx Start Task.vi"("task/channels in"=w338, "error in"=w337) -> ("task out"=w336:refnum<k21>, "error out"=w335:errorcluster)  [unwired: 12 out]
                  }
                }
              }
            }
          }
          frame #1 {
            w357 = 10.0  # timeout (s)
            n163 = local read "Task Name"() -> (w354:refnum<k21>)
            n164 = property class="DAQmx Read"(reference=w354) -> ("AvailSampPerChan"=→"AvailSampPerChan":u32)  [unwired: 1 in, 2 out]
            n165 = call-poly <vilib>:"DAQmx Read.vi"("task/channels in"=w350, "number of samples per channel"="number of samples per channel", "timeout"=w357, "error in"=w349) -> ("data"=w356:waveform(dbl)[])  [unwired: 9 in, 2 out]
            n166 = for {
              tunnel: w356 -> [w376] mode=indexing
              tunnel: [w377] -> _ mode=indexing
              tunnel: [w377] -> w348 mode=indexing
              n167 = call <vilib>:"Mean.vi"("X"=w376) -> ("mean"=w377:dbl)  [unwired: 1 out]
            }
            n168 = local read "Factor A"() -> (w347:dbl[])
            n169 = local read "Factor B"() -> (w346:dbl[])
            n170 = local read "Factor N"() -> (w344:dbl[])
            n171 = for {
              tunnel: w348 -> [w364] mode=indexing
              tunnel: w347 -> [w367] mode=indexing
              tunnel: [w361] -> w339 mode=indexing
              tunnel: w346 -> [w365] mode=indexing
              tunnel: w344 -> [w363] mode=indexing
              n172 = Multiply(x=w364, y=w367) -> (x*y=w366:dbl)
              n173 = Add(x=w366, y=w365) -> (x+y=w362:dbl)
              n174 = Subtract(x=w362, y=w363) -> (x-y=w361:dbl)
            }
            n175 = local read "Offset Nulling"() -> (w345:bool)
            n176 = local read "LVM result file path"() -> (w351:path)
            n177 = local read "Start Recording"() -> (w341:bool)
            n178 = case shown="True" w345 {
              tunnel: w339 -> [_ w359]
              frame False {
              }
              frame True {
                n179 = local write "Factor N"(w359) -> ()
                n180 = local write "Offset Nulling"(FALSE) -> ()
              }
            }
            n181 = local write "Result Array"(w339) -> ()
            n182 = Build Array(w339) -> (w343:dbl[][])
            n183 = local read "Task Name"() -> (w352:refnum<k21>)
            n184 = Index Array(array=w343, index (col)="Display Channel") -> (element=w342:dbl[])  [unwired: 1 in]
            n185 = Transpose 2D Array(2D array=w343) -> (transposed array=w340:dbl[][])
            n186 = local write "Display Channel results"(w342) -> ()
            n187 = case shown="True" w341 {
              tunnel: w351 -> [_ w373]
              tunnel: w340 -> [_ w368]
              tunnel: w352 -> [_ w375]
              tunnel: w343 -> [_ w369]
              frame False {
              }
              frame True {
                n188 = call "Convert to Dynamic Data"("2D Array"=w368) -> ("Dynamic Data Type"=w374:dynamicdata)  [unwired: 3 out]
                n189 = local read "Csv Result File"() -> (w370:path)
                n190 = call "Write To Measurement File"("Signals"=w374, "File Name"=w373, "DAQmx Task"=w375) -> ()  [unwired: 4 in, 13 out]
                n191 = call-poly <vilib>:"Write To Spreadsheet File.vi"("delimiter (\\t)"="," ("delimiter (\\t)"), "append to file? (new file:F)"=TRUE, "2D data"=w369, "file path (dialog if empty)"=w370) -> ()  [unwired: 4 in, 1 out]
              }
            }
          }
          frame #2 {
            n192 = local read "Start Fatigue Module"() -> (w379:bool)
            n193 = case shown="True" w379 {
              tunnel: w378 -> [_ w380]
              frame False {
              }
              frame True {
                n194 = flat-sequence {
                  tunnel: w380 -> [w381]
                  tunnel: w380 -> [w400]
                  frame #0 {
                  }
                  frame #1 {
                    n195 = local read "Channel Name Array"() -> (w388:string[])
                    n196 = Index Array(array=w388, index="Channel to count cycle") -> (element=→"Cycle count measuring":string)
                    n197 = Index Array(array=w381, index="Channel to count cycle") -> (element=w382:dbl)
                    n198 = Greater?(x=w382, y="Upbond") -> (0:w384:bool)
                    n199 = case shown="True" w384 {
                      frame False {
                      }
                      frame True {
                        n200 = local read "Valley"() -> (w390:bool)
                        n201 = case shown="True" w390 {
                          frame False {
                          }
                          frame True {
                            n202 = local write "Valley"(FALSE) -> ()
                            n203 = local read "Current cycle numbers"() -> (w394:dbl)
                            n204 = Add(x=w394, y=1.0) -> (x+y=w393:dbl)
                            n205 = local write "Current cycle numbers"(w393) -> ()
                          }
                        }
                        "Peak" <- TRUE
                      }
                    }
                    n206 = Less?(x=w382, y="Lowerbound") -> (x < y?=w385:bool)
                    n207 = case shown="True" w385 {
                      frame False {
                      }
                      frame True {
                        n208 = local write "Peak"(FALSE) -> ()
                        "Valley" <- TRUE
                      }
                    }
                  }
                  frame #2 {
                    n209 = local read "Current cycle numbers"() -> (w403:dbl)
                    n210 = Quotient & Remainder(x=w403, y="Recording interval (N)") -> (x-y*floor(x/y)=w401:dbl, floor(x/y)=w404:dbl)
                    n211 = Multiply(x=w404, y="Recording interval (N)") -> (x*y=w406:dbl)
                    n212 = Number To Decimal String(number=w406) -> (decimal integer string=w413:string)  [unwired: 1 out]
                    n213 = local read "Working Folder"() -> (w399:string)
                    n214 = Concatenate Strings(w399, "\\" ("string"), "Name of specimen", "_file_" ("string"), w413, ".tdms") -> (w410:string)
                    "concatenated string" <- w410
                    n215 = String To Path(string=w410) -> (path=w411:path)
                    n216 = Less?(x=w401, y=5) -> (x < y?=w412:bool)
                    "Fatigue data recording in progress" <- w412
                    n217 = case shown="True" w412 {
                      tunnel: w411 -> [_ w416]
                      tunnel: w400 -> [_ w415]
                      frame False {
                      }
                      frame True {
                        n218 = call "Convert to Dynamic Data2"("Array"=w415) -> ("Dynamic Data Type"=w414:dynamicdata)  [unwired: 3 in]
                        n219 = call "Write To Measurement File2"("Signals"=w414, "File Name"=w416) -> ()  [unwired: 5 in, 13 out]
                      }
                    }
                  }
                }
              }
            }
          }
        }
      }
    }
  }
